vi "FuncGen.vi"(7 "Enable?":bool, 9 "Frequency [periods/tick]":fxp<+,32,0>, 10 "Amplitude [V]":fxp<+/-,25,5>, 11 "Excitation mode":T1) -> (3 "Output [V]":fxp<+/-,25,5> format="%#.10g")   [LabVIEW 2020, in "ReferenceGen.lvlib"]
doc: "Function generator"
uses:
  ReferenceGen.lvlib
  FPGA TypeDefs/SelectExcitation_Enum.ctl
  <vilib>/Platform/TimedLoop/XDataNode/timing_clust.ctl
  <vilib>/Platform/TimedLoop/XDataNode/nitl_modes.ctl
  <vilib>/Platform/TimedLoop/XDataNode/wakeup.ctl
  <vilib>/rvi/Emulation/niFpgaSctlEmulationGetInTimedLoop.vi
  <vilib>/rvi/Emulation/niFpgaEmulationReportErrorSimple.vi
  <vilib>/rvi/Emulation/niFpgaGetClockAttributes.vi
  <vilib>/rvi/Emulation/niFpgaCriticalErrorInLSC.vi
  <vilib>/Platform/TimedLoop/XDataNode/XDataNode.xnode
  <vilib>/rvi/FXPMathLib/FxpMul/XNode/nifxpmath_Multiplier.xnode
  <vilib>/Platform/TimedLoop/XDataNode/XDNodeRunTimeDep.lvlib
  <vilib>/rvi/FXPMathLib/sim/FxpSim.dll
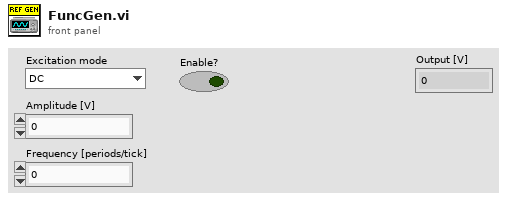
[diagram p1: front panel]
types:
  T1 = typedef "SelectExcitation_Enum.ctl" = enum8{"DC", "Sine", "Square", "WhiteNoise"}
  T2 = typedef "XDNodeRunTimeDep.lvlib/timing_clust.ctl" = cluster{"Expected End [f-1]":u64, "Actual End [f-1]":u64, "Finished Late? [f-1]":bool, "Expected End [i-1]":u64, "Actual End [i-1]":u64, "Finished Late? [i-1]":bool, "Expected Start [i]":u64, "Actual Start [i]":u64, "Expected Start [f]":u64, "Actual Start [f]":u64, "Source Name":string, "Structure Name":string, "Period":i64, "Deadline":i64, "Offset":i64, "Start":i64, "Priority":i32, "Timeout":i32, "Mode":T3, "Wakeup Reason":T4, "Error":errorcluster, "Source Type":string, "Secondary Source Type":string, "Global End Time":u64, "Global Start Time":u64, "Frame Duration":u64, "Iteration Duration":u64, "Assigned CPU":i32, "I/O Scan Engine Mode":u32}
  T3 = typedef "XDNodeRunTimeDep.lvlib/nitl_modes.ctl" = enum32{"No Change", "Process missed periods, maintain original phase", "Discard missed periods, maintain original phase", "Process missed periods, ignore original phase", "Discard missed periods, ignore original phase"}
  T4 = typedef "XDNodeRunTimeDep.lvlib/wakeup.ctl" = enum32{"Normal", "Aborted", "Asynchronous wakeup", "Timing source error", "Timed loop error", "Timeout"}
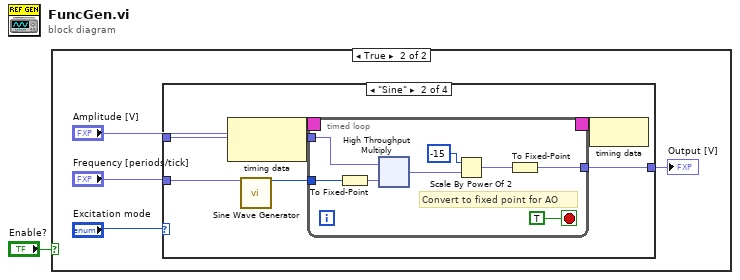
[diagram p0: block diagram]
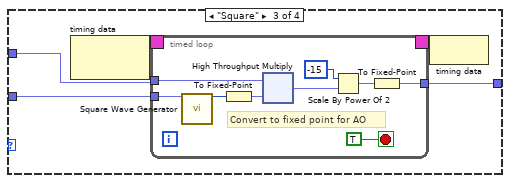
[diagram p4: hidden frame]
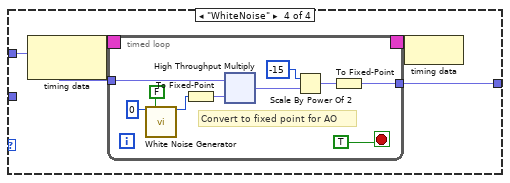
[diagram p5: hidden frame]
diagram:
  n1 = case shown="True" "Enable?" {
    frame False {
    }
    frame True {
      n2 = case shown="\"Sine\"" "Excitation mode" {
        tunnel: "Amplitude [V]" -> [w6 w11 w28 w46]
        tunnel: [w6 w10 w27 w45] -> w2
        tunnel: "Frequency [periods/tick]" -> [_ w9 w29 _]
        frame "DC", Default {
        }
        frame "Sine" {
          n3 = node-c288() -> (w8:T2)  [unwired: 1 in]
          n4 = call "Sine Wave Generator"("frequency (periods/tick)"=w9) -> ("sine out"=w12:i16)  [unwired: 14 in]
          n5 = timed-loop {
            timing: w8 -> [_]
            timing-out: [_] -> w7
            tunnel: w12 -> [w19]
            tunnel: w11 -> [w18]
            tunnel: [w13] -> w10
            stop <- TRUE stop-if-true
            # "Convert to fixed point for AO"
            n6 = To Fixed-Point(number=w19) -> (fixed-point=w20:fxp<+/-,16,16>)  [unwired: 1 in]
            n7 = xnode ("High Throughput Multiply")("x"=w18, "y"=w20) -> ("x*y"=w15:fxp<+/-,41,21>)
            n8 = Scale By Power Of 2(n=i16 -15, x=w15) -> (x*2^n=w14:fxp<+/-,41,21>)
            n9 = To Fixed-Point(number=w14) -> (fixed-point=w13:fxp<+/-,25,5>)  [unwired: 1 in]
          }
          n10 = node-c288(w7) -> ()
        }
        frame "Square" {
          n11 = node-c288() -> (w26:T2)  [unwired: 1 in]
          n12 = timed-loop {
            timing: w26 -> [_]
            timing-out: [_] -> w25
            tunnel: w29 -> [w38]
            tunnel: w28 -> [w33]
            tunnel: [w30] -> w27
            stop <- TRUE stop-if-true
            # "Convert to fixed point for AO"
            n13 = call "Square Wave Generator"("frequency (periods/tick)"=w38) -> ("square wave out"=w34:i16)  [unwired: 14 in]
            n14 = To Fixed-Point(number=w34) -> (fixed-point=w37:fxp<+/-,16,16>)  [unwired: 1 in]
            n15 = xnode ("High Throughput Multiply")("x"=w33, "y"=w37) -> ("x*y"=w36:fxp<+/-,41,21>)
            n16 = Scale By Power Of 2(n=i16 -15, x=w36) -> (x*2^n=w31:fxp<+/-,41,21>)
            n17 = To Fixed-Point(number=w31) -> (fixed-point=w30:fxp<+/-,25,5>)  [unwired: 1 in]
          }
          n18 = node-c288(w25) -> ()
        }
        frame "WhiteNoise" {
          n19 = node-c288() -> (w44:T2)  [unwired: 1 in]
          n20 = timed-loop {
            timing: w44 -> [_]
            timing-out: [_] -> w43
            tunnel: w46 -> [w52]
            tunnel: [w47] -> w45
            stop <- TRUE stop-if-true
            # "Convert to fixed point for AO"
            n21 = call "White Noise Generator"("seed"=u32 0, "reset"=FALSE) -> ("white noise out"=w53:i16)  [unwired: 13 in]
            n22 = To Fixed-Point(number=w53) -> (fixed-point=w56:fxp<+/-,16,16>)  [unwired: 1 in]
            n23 = xnode ("High Throughput Multiply")("x"=w52, "y"=w56) -> ("x*y"=w55:fxp<+/-,41,21>)
            n24 = Scale By Power Of 2(n=i16 -15, x=w55) -> (x*2^n=w48:fxp<+/-,41,21>)
            n25 = To Fixed-Point(number=w48) -> (fixed-point=w47:fxp<+/-,25,5>)  [unwired: 1 in]
          }
          n26 = node-c288(w43) -> ()
        }
      }
      "Output [V]" <- w2
    }
  }
